vi "SubPanel_DataCollection_Rev11_v16.vi"(0 "DCPowerInformationClusterArray_Input":T8(array[cluster]), 1 "VISAPowerInfoInputArray":T5(array[cluster]), 2 "Run Data SubPanel Input":T4, 3 "RF Block Input Array":T3[](array[typedef]), 4 "Oscilloscope Info Array":T7(array[cluster]) {"vertical coupling" items=["AC", "DC", "Ground"]}, 5 "Plot Color Array":u32[](array[colorbox])=[16711686, 65351, 8978420, 14474240, 16139007, 16752640, 8958719, 16758973, 16777215, 46792, 11992992, 12961221, 16763690, 12600063, 16711835, 2953983, 40796, 13111296, 13352613, 9221011, 12964076, 12819897, 65442, 16776704, 14540253, 16740729, 10658047, 10813344, 16753521, 13413843, 8691115, 10339240, 14401205, 16746704, 7467519, 16775978, 13872558, 11387603, 13354405, 10420227, 13107364, 4060, 35208, 11817216, 7566080, 40796, 7539456, 2837073, 6372186, 7499083, 10648702, 16757152], 6 "New Run?":bool, 7 "error in":errorcluster) -> (20 "DCPowerInformationClusterArray_Output":T8(array[cluster]), 21 "VISAPowerInfoInputOutput":T5(array[cluster]), 22 "Run Data SubPanel Output":T4, 23 "RF Subpanel Output":T3[](array[typedef]), 24 "Oscilloscope Info Array":T7(array[cluster]) {"vertical coupling" items=["AC", "DC", "Ground"]}, 25 "Reinitialize?":bool, 26 "Data Was Collected?":bool, 27 "error out":errorcluster)   [LabVIEW 2019]
uses:
  Controls/DataBlockControl.ctl
  Controls/QueueDataControl_V3.ctl
  <vilib>/Utility/file.llb/Write Delimited Spreadsheet (string).vi
  <instrlib>/niScope/Acquire/Fetch/niScope Multi Fetch Binary 16.vi
  Controls/RFBlockControl.ctl
  <instrlib>/niScope/Controls/niScope vertical coupling.ctl
panel:
  out "wfm":i16[][](array[numeric])
  in  "Total Time X Min":dbl
  in  "Total Time X Max":dbl
  in  "Total Current Y Min":dbl
  in  "Total Current Y Max":dbl
  in  "Total Voltage Y Min":dbl
  in  "Total Voltage Y Max":dbl
  in  "Total Measurement Range Update":bool
  in  "Device Powered?":bool=TRUE
  out "output cluster":T2 {"vertical coupling" items=["AC", "DC", "Ground"]}
  in  "Live Measurement Range Update":bool
  in  "Live Current Y Min":dbl
  in  "Live Current Y Max":dbl
  in  "Live Voltage Y Min":dbl
  in  "Live Voltage Y Max":dbl
  out "Current Measurements Live":cluster{dbl[], dbl[]}[](graph)
  out "Voltage Measurements Live":cluster{dbl[], dbl[]}[](graph)
  out "Voltage Waveform Array":waveform(dbl)[](graph)
  out "Current Waveform Array":waveform(dbl)[](graph)
  out "Current Measurements Total":cluster{dbl[], dbl[]}[](graph)
  out "Voltage Measurements Total":cluster{dbl[], dbl[]}[](graph)
  out "Exiting":bool
  out "Full Run Information":string
  out "Ready For Next Run?":bool
  in  "Next Run":bool
  out "Recording Data":bool
  in  "Record Data Toggle":bool
  out "error of collection":errorcluster
  in  "force exit SubVI":bool
  out "RF Block Parameters Output":T3
  in  "Oscilloscope Info Array":T6(array[cluster]) {"vertical coupling" items=["AC", "DC", "Ground"]}
  out "seconds since 1Jan1904 2":timestamp
  out "seconds since 1Jan1904":timestamp
  out "Numeric 2":i32
  out "Numeric":i32
  out "RFSourceInfoArray":string[][](array[string])
  out "OscilloscopeInfoArray":string[][](array[string])
  out "DCPowerInfoArray":string[][](array[string])
  # "Background information (Important)\nThere are three sets of voltage/current graphs\n\nOne is live always and just shows what all the channels look like _______ Waveform Array\n\nOne is live when measuring and shows some duration of the recording _______ Measurements Live\n\nOne shows the entire duration of the run, but it will take a few seconds to compile, just be patient it will populate\n\n\nInstructions (More Important)"
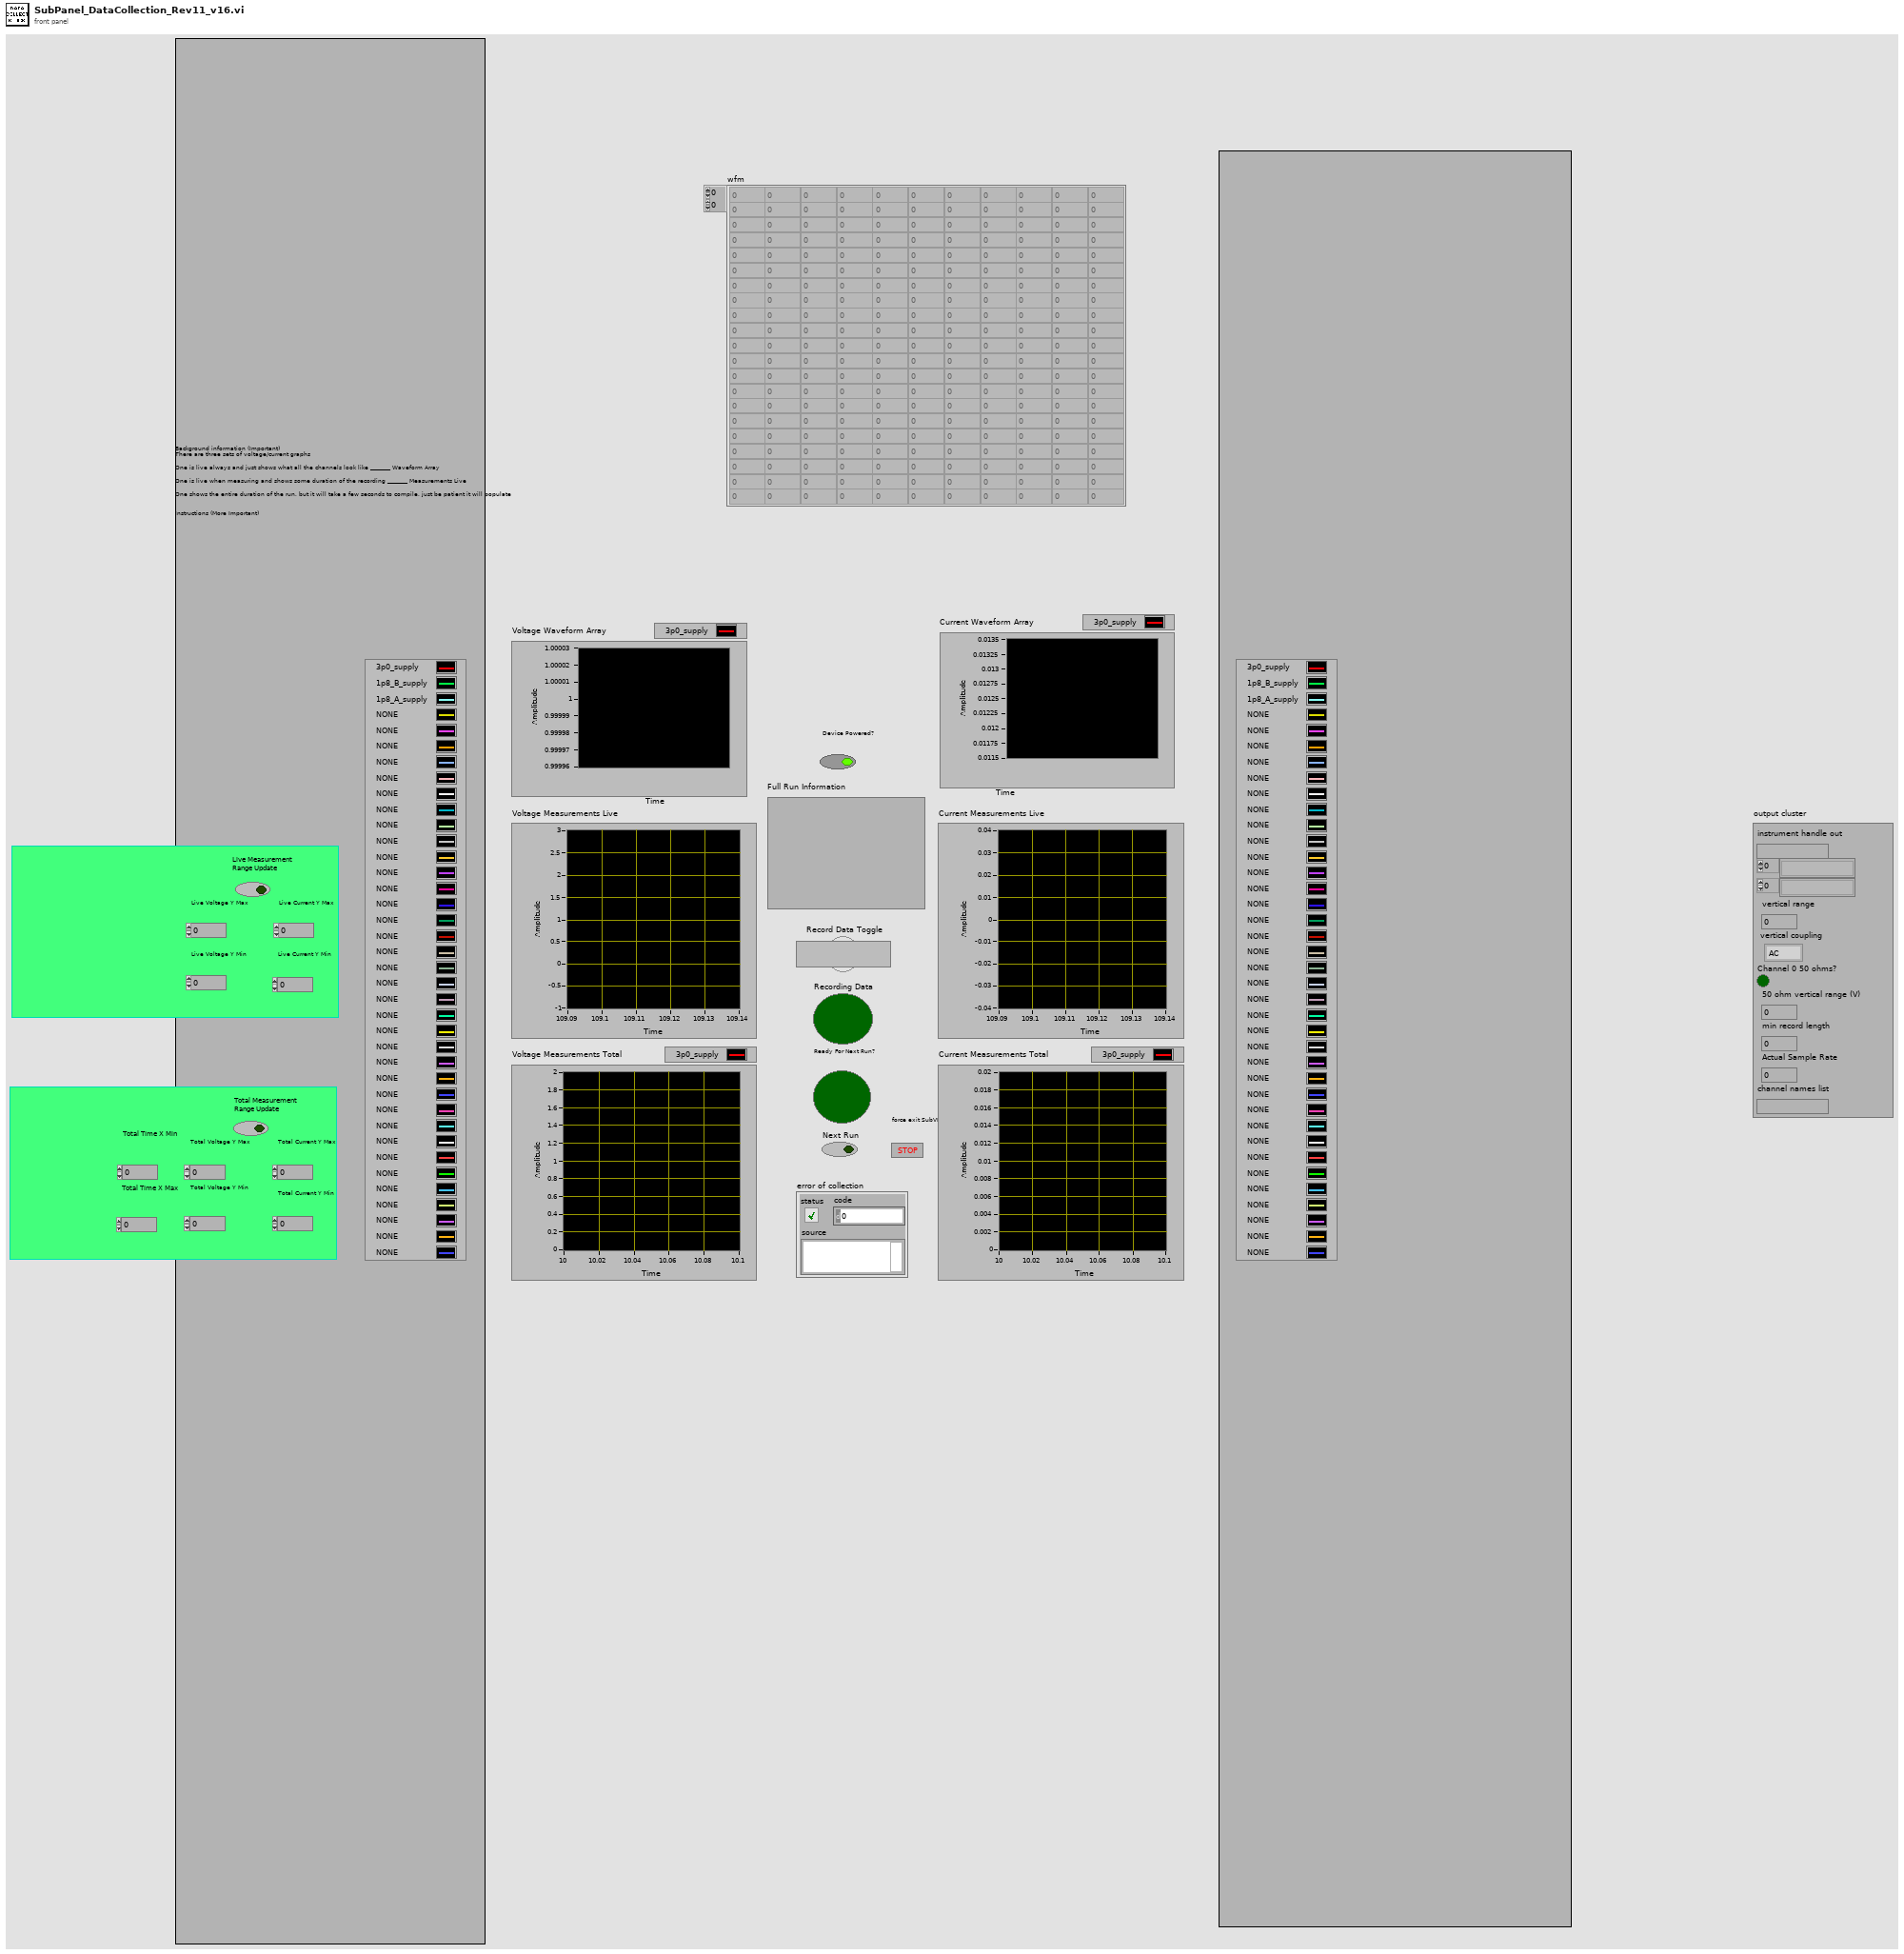
[diagram p1: front panel]
types:
  T1 = typedef "niScope vertical coupling.ctl" = i32
  T2 = cluster{"instrument handle out":refnum<k15>, string[], string[], "vertical range":dbl, "vertical coupling":T1, "Channel 0 50 ohms?":bool, "50 ohm vertical range (V)":dbl, "min record length":i32, "Actual Sample Rate":dbl, "channel names list":string}
  T3 = typedef "RFBlockControl.ctl" = cluster{"VISA resource name":refnum<visa-resource-name>, "RF Power State In":bool, "Frequency (GHz) Output":dbl, "Power (dBm) Output":dbl, "Instrument Name":string}
  T4 = typedef "DataBlockControl.ctl" = cluster{"Run Folder Parent Directory":path, "DUT":string, "Ion (ex Kr)":string, "Board Number":string, "Effective LET":string, "Test Type":enum16{"Single Event Latchup", "Single Event Transient", "Single Event Upset"}}
  T5 = cluster{"VISA resource name":refnum<visa-resource-name>, "String List":string, string[], "Input Array (Voltage,Current_Limit)":dbl[], "Input Array (Voltage,Current_Limit)":dbl[], "Channel Names":string[], "read buffer":string}[]
  T6 = cluster{"instrument handle out":refnum<k15>, "channel numbers array":string[], "channel names array":string[], "vertical range":dbl, "vertical coupling":T1, "Channel 0 50 ohms?":bool, "50 ohm vertical range (V)":dbl, "min record length":i32, "Actual Sample Rate":dbl}[]
  T7 = cluster{"instrument handle out":refnum<k15>, string[], string[], "vertical range":dbl, "vertical coupling":T1, "Channel 0 50 ohms?":bool, "50 ohm vertical range (V)":dbl, "min record length":i32, "Actual Sample Rate":dbl, "channel names list":string}[]
  T8 = cluster{"IVI Refnum out":refnum<k15>, "Active Channel Numbers String List":string, "Active Channel Numbers Array":string[], "Active Channel Voltage Array":dbl[], "Active Channel Names Array":string[], "Active Channel Current Limit Array":dbl[], "Active Channel Measure Record Delta Time Array":dbl[], "All Channel Numbers Array":string[]}[]
  T9 = typedef "QueueDataControl_V3.ctl" = cluster{"Array of fetched data":dbl[][][], "Channel Names Array":string[], "Voltage Waveform Array":waveform(dbl)[], "Current Waveform Array":waveform(dbl)[], "Resetting Time":timestamp, "Beam Logic":dbl}
  T10 = cluster{"IVI Refnum out":refnum<k15>, string, "voltage level channel 23":dbl, "Channel Name 23":string, "Current Limit":dbl, "Measure Record dt":dbl, string, "Current Threshold Reset Value Array":dbl}[]
  T11 = cluster{timestamp[], "wfm info":cluster{"actualSamples":i32, "absoluteInitialX":dbl, "relativeInitialX":dbl, "xIncrement":dbl, "offset":dbl, "gain":dbl, "reserved1":dbl, "reserved2":dbl}[][], "wfm":i16[][][]}
  T12 = cluster{"actualSamples":i32, "absoluteInitialX":dbl, "relativeInitialX":dbl, "xIncrement":dbl, "offset":dbl, "gain":dbl, "reserved1":dbl, "reserved2":dbl}[]
  T13 = cluster{"created path array":path[], "DCPowerInformationArrayOutput":cluster{"IVI Refnum out":refnum<k15>, string, "voltage level channel 23":dbl, "Channel Name 23":string, "Current Limit":dbl, "Measure Record dt":dbl, string, "Current Threshold Reset Value Array":dbl}[], string[]}
  T14 = cluster{"Array of fetched data":dbl[][], string, i32[]}
  T15 = enum16{"open", "replace", "create", "open or create", "replace or create", "replace or create with confirmation"}
  T16 = enum16{"Single Event Latchup", "Single Event Transient", "Single Event Upset"}
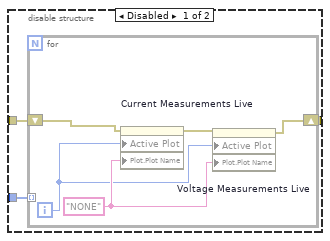
[diagram p2: hidden frame]
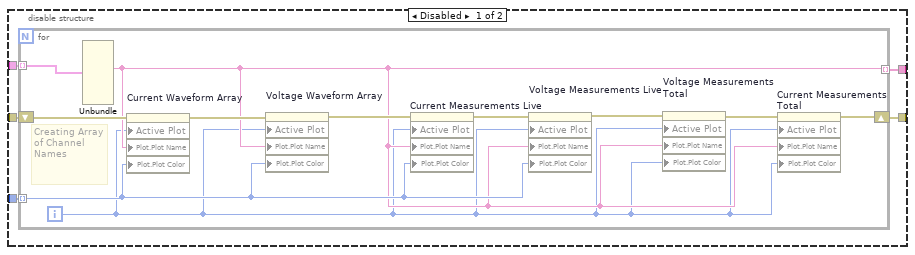
[diagram p3: hidden frame]
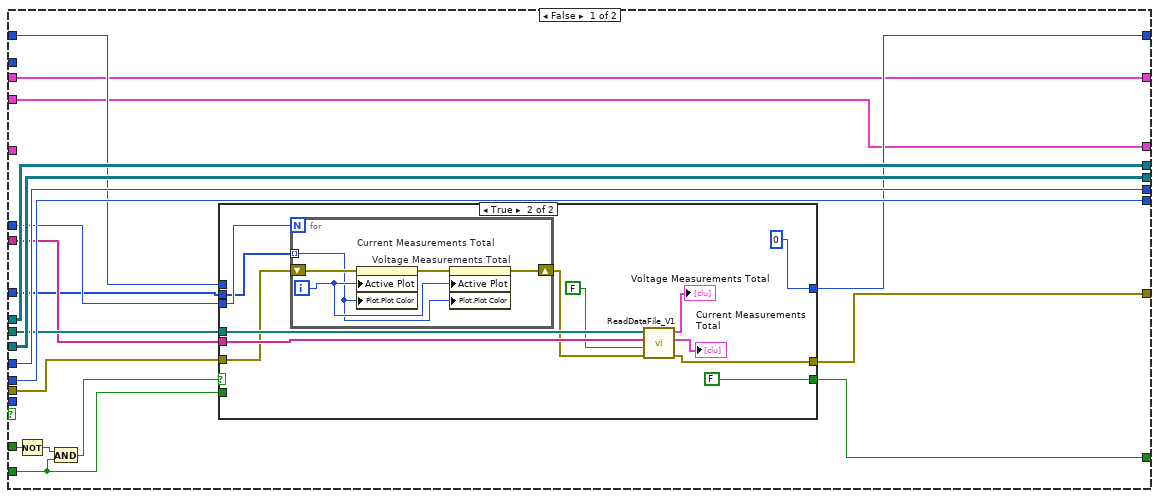
[diagram p11: hidden frame]
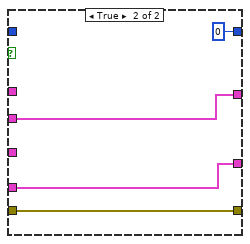
[diagram p13: hidden frame]
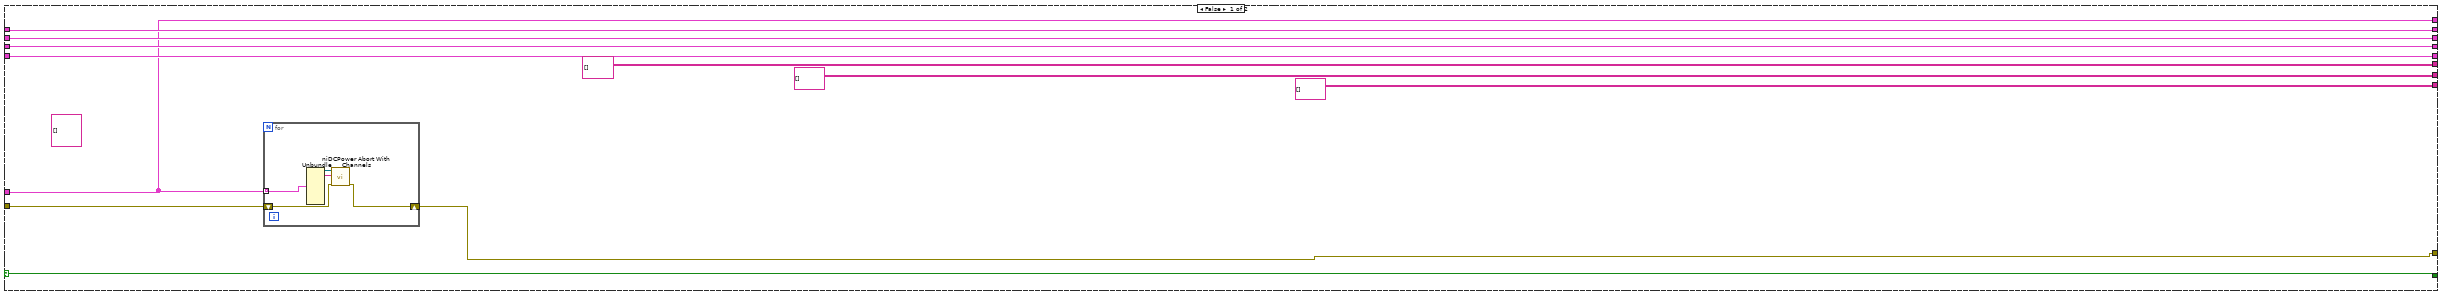
[diagram p14: hidden frame]
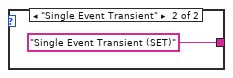
[diagram p15: hidden frame]
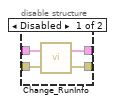
[diagram p19: hidden frame]
diagram:
  w25 = cluster{dbl[], dbl[]}[] [] ("array")
  (unwired) string[] ["Instrument Name", "Channel Name", "Instrument Channel Number", "Voltage (V)", "Current Limit (A)", "Measure Record delta Time (s)"] ("new element/subarray")
  w55 = T9 {"Array of fetched data"=[], "Channel Names Array"=[], "Voltage Waveform Array"=[], "Current Waveform Array"=[], "Resetting Time"=timestamp(0 s since 1904-01-01), "Beam Logic"=0.0} ("DCPower Queue Data Double Array Format")
  (unwired) T9 {"Array of fetched data"=[], "Channel Names Array"=[], "Voltage Waveform Array"=[], "Current Waveform Array"=[], "Resetting Time"=timestamp(0 s since 1904-01-01), "Beam Logic"=0.0} ("DCPower Double Array Queue")
  (unwired) 10000 ("binary file indexor in")
  (unwired) T4 {"Run Folder Parent Directory"=path "", "DUT"="", "Ion (ex Kr)"="", "Board Number"="", "Effective LET"="", "Test Type"=enum."Single Event Latchup"} ("Run Data Configuration")
  # "A flag to state if the devices are powered on or off"
  # "Need to make a function that will decrease the amount of loops if there are more channels active. Just exponential decay or a X/Y function but need some kind of offset which will probably be experimentally determined"
  # "Initiating the queue"
  # "echoing run information"
  # "Checking if this is a new run. If it is, a new folder is created along with references to a datafile node. If it is not new (i.e. you didn't start recording data because you needed to make a last minute change and pressed forced exit subvi), the previous folder that is theoretically empty (or just has the .txt files is used"
  # "If yes, you go into this subVI"
  # "This is the message at the beginning confirming if you want to make small changes to the program (i.e. LET)"
  # "Parameters from the configuration stage of this program"
  # "Reset the graph that is saving every 10 seconds of data. Every reset the low bound of the ten seconds is"
  # "Need to change to reflect number of channels that are being recorded. Collect this from a parameters file eventually that will be created"
  # "Indicator if the system is ready for another run. Also indicates if data was actually collected"
  # "Resets the system to start recording"
  # "A flag to ensure the warning message shows only once and doesn't lock the system"
  # "Initiating all of the DC Power instruments (doing this here so because we force abort channels in the DCPower setup because buffer overflow issues. Iterating over the instrument array and the active channel list"
  n1 = flat-sequence {
    tunnel: [w94] -> w71
    tunnel: "error in" -> [w84]
    tunnel: [w98] -> w76
    tunnel: "Run Data SubPanel Input" -> [w86]
    frame #0 {
      n2 = disable-structure shown="Enabled" {
        disable-tunnel: w84 -> [w101 w112]
        disable-tunnel: [w110 w112] -> w83
        frame Enabled {
          n3 = property on="Voltage Measurements Live" class="XYGraph (strict)"(error in=w101, "BG Color"=u32 0 ("Plot.Plot Color"), "Plot.Plot Interpolation"=u8 2) -> (error out=w100:errorcluster)  [unwired: 1 in, 1 out]
          n4 = property on="Current Measurements Live" class="XYGraph (strict)"(error in=w100, "BG Color"=u32 0 ("Plot.Plot Color"), "Plot.Plot Interpolation"=u8 2) -> (error out=w99:errorcluster)  [unwired: 1 in, 1 out]
          n5 = property on="Voltage Measurements Total" class="XYGraph (strict)"(error in=w99, "BG Color"=u32 0 ("Plot.Plot Color"), "Plot.Plot Interpolation"=u8 2) -> (error out=w111:errorcluster)  [unwired: 1 in, 1 out]
          n6 = property on="Current Measurements Total" class="XYGraph (strict)"(error in=w111, "BG Color"=u32 0 ("Plot.Plot Color"), "Plot.Plot Interpolation"=u8 2) -> (error out=w110:errorcluster)  [unwired: 1 in, 1 out]
        }
        frame Disabled {
        }
      }
      n7 = local write "Voltage Measurements Total"(cluster{dbl[], dbl[]}[] [] ("Voltage Measurements")) -> ()
      n8 = local write "Current Measurements Total"(cluster{dbl[], dbl[]}[] [] ("Current Measurements")) -> ()
      n9 = local write "Recording Data"(FALSE ("Recording Data")) -> ()
      n10 = local write "Exiting"(FALSE ("Forced Exit")) -> ()
      n11 = call "Convert_RunInfoCluster_2_RunInfoStringList.vi"("error in"=w83, "Run Number"="", "Run Data SubPanel Input"=w86) -> ("error output"=w87:errorcluster, "Run Data Output"=w88:string)
      n12 = call "Display Message to User"("error in (no error)"=w87, "Enable"=TRUE, "Message"=w88) -> ("error out"=w94:errorcluster)  [unwired: 7 in, 1 out]
      n13 = Two Button Dialog(message="Changing the LET?", 1:"No" ("F button name (\"Cancel\")"), 2:"Yes" ("T button name (\"OK\")")) -> (T button?=w98:bool)
    }
  }
  n14 = call "Convert_InstrumentReferenceArray_2_ChannelReferenceArray.vi"("error in (no error)"=w71, "DCPowerInformationClusterArray_Input"="DCPowerInformationClusterArray_Input") -> ("error out"=w70:errorcluster, "DCPowerInformationArrayOutput"=w20:T10)
  n15 = case shown="True" w76 {
    tunnel: "Run Data SubPanel Input" -> [w114 w118]
    tunnel: [w114 w117] -> w33
    tunnel: [w113 w116] -> w72
    tunnel: w70 -> [w113 w115]
    frame False {
    }
    frame True {
      n16 = disable-structure shown="Enabled" {
        disable-tunnel: w118 -> [w122 w124]
        disable-tunnel: [w121 w123] -> w117
        disable-tunnel: [w120 w126] -> w116
        disable-tunnel: w115 -> [w119 w125]
        frame Disabled {
          n17 = call "Change_RunInfo.vi"("error in (no error)"=w119, "Run Data SubPanel in"=w122) -> ("error out"=w120:errorcluster, "Run Data SubPanel out"=w121:T4)
        }
        frame Enabled {
          n18 = call "Change_RunInfo_V2.vi"("error in (no error)"=w125, "Run Data SubPanel in"=w124) -> ("error out"=w126:errorcluster, "Run Data SubPanel out"=w123:T4)
        }
      }
    }
  }
  n19 = Unbundle(w33) -> ("Run Folder Parent Directory"=w73:path)  [unwired: 5 out]
  n20 = List Folder(path=w73, error in=w72) -> (folder names=w74:string[], error out=w58:errorcluster)  [unwired: 2 in, 2 out]
  n21 = Array Size(array=w74) -> (size(s)=w61:i32)
  n22 = case shown="True" "New Run?" {
    selector: "New Run?" -> [w128 w131]
    tunnel: [w129 w133] -> w62
    tunnel: w61 -> [w129 w132]
    tunnel: [w128 w131] -> w60
    tunnel: [w127 w130] -> w59
    tunnel: w58 -> [w127 w130]
    frame False {
    }
    frame True {
      n23 = Increment(x=w132) -> (x+1=w133:i32)
    }
  }
  n24 = Number To Decimal String(number=w62) -> (decimal integer string=w65:string)  [unwired: 1 in]
  n25 = Concatenate Strings("Run_", w65) -> (w32:string)
  n26 = Array Size(array=w20) -> (size(s)=w57:i32)
  n27 = call "InitialFileFolderCreation_V2.vi"("New Run?"=w60, "error in (no error)"=w59, "Run Number"=w32, "Subfolders&NumChannelsRecorded"=w57, "base path"=w73) -> ("error out"=w31:errorcluster, "SupplementalDataFileReferenceObjectArrayWsubfolders"=w68:refnum<file>[][], "DataFileReferenceObjectArrayWsubfolders"=w69:refnum<file>[][], "created path array"=w36:path[])  [unwired: 3 in]
  n28 = call "Convert_RunInfoCluster_2_RunInfoStringList.vi"("error in"=w31, "Run Number"=w32, "Run Data SubPanel Input"=w33) -> ("error output"=w30:errorcluster, "Run Data Output"=→"Full Run Information":string)
  n29 = for {
    shift-right: [w134] -> w17
    shift-left: w30 -> [w136]
    tunnel: "DCPowerInformationClusterArray_Input" -> [w138] mode=indexing
    n30 = Unbundle(w138) -> ("IVI Refnum out"=w135:refnum<k15>, "Active Channel Numbers String List"=w137:string)  [unwired: 6 out]
    n31 = call <instrlib>:"niDCPower Initiate With Channels.vi"("error in (no error)"=w136, "channel name"=w137, "instrument handle"=w135) -> ("error out"=w134:errorcluster)  [unwired: 7 in, 1 out]
  }
  n32 = disable-structure shown="Enabled" {
    disable-tunnel: "Plot Color Array" -> [w141 _]
    disable-tunnel: [w140 w147] -> w18
    disable-tunnel: w17 -> [w139 w147]
    frame Disabled {
      n33 = for {
        shift-right: [w144] -> w140
        shift-left: w139 -> [w146]
        tunnel: w141 -> [_] mode=indexing
        i -> [w142]
        w143 = "NONE" ("Plot.Plot Name")
        n34 = property on="Current Measurements Live" class="XYGraph (strict)"(error in=w146, "Active Plot"=w142, "Plot.Plot Name"=w143) -> (error out=w145:errorcluster)  [unwired: 1 in, 1 out]
        n35 = property on="Voltage Measurements Live" class="XYGraph (strict)"(error in=w145, "Active Plot"=w142, "Plot.Plot Name"=w143) -> (error out=w144:errorcluster)  [unwired: 1 in, 1 out]
      }
    }
    frame Enabled {
    }
  }
  n36 = case shown="Error .." w18 {
    selector: w18 -> [w148 _]
    tunnel: [w148 w149] -> w3
    tunnel: w17 -> [_ w149]
    frame No Error {
    }
    frame Error {
    }
  }
  n37 = disable-structure shown="Enabled" {
    disable-tunnel: [w154 w167] -> w21
    disable-tunnel: w20 -> [w153 w168]
    disable-tunnel: "Plot Color Array" -> [w152 _]
    disable-tunnel: [w151 w166] -> w4
    disable-tunnel: w3 -> [w150 w166]
    frame Disabled {
      n38 = for {
        tunnel: w153 -> [w164] mode=indexing
        tunnel: [w156] -> w154 mode=indexing
        shift-right: [w157] -> w151
        shift-left: w150 -> [w161]
        tunnel: w152 -> [w160] mode=indexing
        i -> [w155]
        # "Creating Array of Channel Names"
        n39 = Unbundle(w164) -> ("Channel Name 23"=w156:string)  [unwired: 7 out]
        n40 = property on="Current Waveform Array" class="WFChart (strict)"(error in=w161, "Active Plot"=w155, "Plot.Plot Name"=w156, "Plot.Plot Color"=w160) -> (error out=w163:errorcluster)  [unwired: 1 in, 1 out]
        n41 = property on="Voltage Waveform Array" class="WFChart (strict)"(error in=w163, "Active Plot"=w155, "Plot.Plot Name"=w156, "Plot.Plot Color"=w160) -> (error out=w162:errorcluster)  [unwired: 1 in, 1 out]
        n42 = property on="Current Measurements Live" class="XYGraph (strict)"(error in=w162, "Active Plot"=w155, "Plot.Plot Name"=w156, "Plot.Plot Color"=w160) -> (error out=w165:errorcluster)  [unwired: 1 in, 1 out]
        n43 = property on="Voltage Measurements Live" class="XYGraph (strict)"(error in=w165, "Active Plot"=w155, "Plot.Plot Name"=w156, "Plot.Plot Color"=w160) -> (error out=w159:errorcluster)  [unwired: 1 in, 1 out]
        n44 = property on="Voltage Measurements Total" class="XYGraph (strict)"(error in=w159, "Active Plot"=w155, "Plot.Plot Name"=w156, "Plot.Plot Color"=w155) -> (error out=w158:errorcluster)  [unwired: 1 in, 1 out]
        n45 = property on="Current Measurements Total" class="XYGraph (strict)"(error in=w158, "Active Plot"=w155, "Plot.Plot Name"=w156, "Plot.Plot Color"=w155) -> (error out=w157:errorcluster)  [unwired: 1 in, 1 out]
      }
    }
    frame Enabled {
      n46 = for {
        tunnel: w168 -> [w170] mode=indexing
        tunnel: [w169] -> w167 mode=indexing
        n47 = Unbundle(w170) -> ("Channel Name 23"=w169:string)  [unwired: 7 out]
      }
    }
  }
  n48 = case shown="Error .." w4 {
    selector: w4 -> [w171 _]
    tunnel: [w171 w172] -> w2
    tunnel: w3 -> [_ w172]
    frame No Error {
    }
    frame Error {
    }
  }
  n49 = disable-structure shown="Enabled" {
    disable-tunnel: w2 -> [w176 w178]
    disable-tunnel: [w175 w178] -> w7
    disable-tunnel: [w174 _] -> w22
    disable-tunnel: w55 -> [w173 _]
    frame Enabled {
      n50 = Obtain Queue(name (unnamed)="DCPowerQueue", element data type=w173, error in (no error)=w176) -> (queue out=w174:refnum<queue>, error out=w175:errorcluster)  [unwired: 2 in, 1 out]
    }
    frame Disabled {
    }
  }
  n51 = disable-structure shown="Enabled" {
    disable-tunnel: "Oscilloscope Info Array" -> [w183 _]
    disable-tunnel: [w180 w235] -> w10
    disable-tunnel: w7 -> [w184 w235]
    frame Enabled {
      w186 = T11 {[], "wfm info"=[], "wfm"=[]} ("output cluster")
      n52 = for {
        tunnel: w183 -> [w195] mode=indexing
        shift-right: [w197] -> w185
        shift-left: w184 -> [w196]
        n53 = Unbundle By Name(w195) -> ("instrument handle out"=w194:refnum<k15>)
        n54 = call <instrlib>:"niScope Initiate Acquisition.vi"("instrument handle"=w194, "error in"=w196) -> ("error out"=w197:errorcluster)  [unwired: 12 in, 1 out]
      }
      n55 = Obtain Queue(name (unnamed)="OscilloscopeDataQueue", element data type=w186, error in (no error)=w185) -> (queue out=w187:refnum<queue>, error out=w189:errorcluster)  [unwired: 2 in, 1 out]
      n56 = while {
        shift-right: [w206] -> w181
        shift-left: w189 -> [w209]
        shift-right: [w207] -> w179
        shift-left: w183 -> [w207]
        tunnel: w187 -> [_]
        tunnel: w186 -> [w208]
        tunnel: [w205] -> _
        shift-right: [w199] -> _
        shift-left: FALSE ("x") -> [w200]
        i -> [w198]
        stop <- w204 stop-if-true
        # "BASE OFF OF TAMU POWER SCRIPTS"
        n57 = for {
          tunnel: w207 -> [w215] mode=indexing
          shift-right: [w223] -> w206
          shift-left: w209 -> [w219]
          tunnel: [w222] -> w202 mode=indexing
          tunnel: [w221] -> w201 mode=indexing
          tunnel: [w210] -> w203 mode=indexing
          shift-right: [w216] -> w199
          shift-left: w200 -> [w213]
          tunnel: w198 -> [w214]
          tunnel: w198 -> [w211]
          i -> [w220]
          n58 = Get Date/Time In Seconds() -> (seconds since 1Jan1904=w210:timestamp)
          n59 = Not(x=w213) -> (.not. x?=w218:bool)
          n60 = Unbundle By Name(w215) -> ("instrument handle out"=w227:refnum<k15>, "channel names list"=w225:string)
          n61 = And(x=w219, y=w218) -> (x .and. y?=w217:bool)
          n62 = Equal To 0?(x=w211) -> (x = 0?=w212:bool)
          n63 = case shown="True" w217 {
            tunnel: w220 -> [_ w234]
            tunnel: [w229 TRUE] -> w216
            tunnel: w215 -> [_ w233]
            tunnel: w214 -> [_ w232]
            tunnel: w213 -> [w229 _]
            tunnel: w210 -> [_ w230]
            frame False {
            }
            frame True {
              "Numeric" <- w234
              "output cluster" <- w233
              "Numeric 2" <- w232
              "seconds since 1Jan1904" <- w230
            }
          }
          n64 = case shown="True" w212 {
            tunnel: w210 -> [_ w228]
            frame False {
            }
            frame True {
              "seconds since 1Jan1904 2" <- w228
            }
          }
          n65 = call-poly <instrlib>:"niScope Fetch (poly).vi"("timeout"=0.0, "error in"=w219, "numSamples"=-1, "channels"=w225, "instrument handle"=w227) -> ("error out"=w223:errorcluster, "wfm"=w221:i16[][], "wfm info"=w222:T12)  [unwired: 3 in, 1 out]
          "wfm" <- w221
        }
        n66 = Bundle(cluster=w208, w203, "wfm info"=w202, "wfm"=w201) -> (w205:T11)
        n67 = local read "Exiting"() -> (w204:bool)
      }
      n68 = for {
        shift-right: [w192] -> w180
        shift-left: w181 -> [w193]
        tunnel: w179 -> [w191] mode=indexing
        n69 = Unbundle By Name(w191) -> ("instrument handle out"=w190:refnum<k15>)
        n70 = call <instrlib>:"niScope Abort.vi"("instrument handle"=w190, "error in"=w193) -> ("error out"=w192:errorcluster)  [unwired: 12 in, 1 out]
      }
    }
    frame Disabled {
      # "get the 1355 board"
    }
  }
  n71 = Bundle("created path array"=w36, "DCPowerInformationArrayOutput"=w20, w21) -> (w48:T13)  [unwired: 1 in]
  n72 = Array Size(array=w21) -> (size(s)=w24:i32)
  n73 = Get Date/Time In Seconds() -> (seconds since 1Jan1904=w35:timestamp)
  n74 = while {
    shift-right: [w271] -> w40
    shift-left: "DCPowerInformationClusterArray_Input" -> [w271]
    shift-right: [w275] -> w41
    shift-left: "VISAPowerInfoInputArray" -> [w275]
    shift-right: [w274] -> w43
    shift-left: w33 -> [w274]
    shift-right: [w273] -> w45
    shift-left: "RF Block Input Array" -> [w273]
    shift-right: [w272] -> w47
    shift-left: "Oscilloscope Info Array" -> [w272]
    shift-right: [w243] -> w56
    shift-left: w7 -> [w270]
    tunnel: w20 -> [w240]
    shift-right: [w269] -> _
    shift-left: FALSE -> [w266]
    tunnel: w22 -> [w268]
    shift-right: [w253] -> _
    shift-left: FALSE -> [w258]
    tunnel: [w262] -> w80
    shift-right: [w256] -> _
    shift-left: TRUE ("x .and. y?") -> [w257]
    shift-right: [w254] -> _
    shift-left: w35 -> [w255]
    tunnel: [w253] -> w39
    tunnel: w55 -> [w251]
    shift-right: [w248] -> w14
    shift-left: timestamp(0 s since 1904-01-01) ("seconds since 1Jan1904") -> [w247]
    shift-right: [w237] -> _
    shift-left: TRUE -> [w236]
    stop <- w252 stop-if-true
    # "If I am going to reset the entire configuration or if we are going up in LET only. True, reset the system. False, don't reset the system"
    n75 = Not(x=w258) -> (.not. x?=w260:bool)
    n76 = And(x="Record Data Toggle", y=w260) -> (x .and. y?=w261:bool)
    "Recording Data" <- w261
    n77 = case shown="False" w261 {
      tunnel: w240 -> [w343 w358]
      tunnel: w270 -> [w341 w365]
      tunnel: [w331 w353] -> w250
      tunnel: [w332 w352] -> w249
      tunnel: w266 -> [_ w363]
      tunnel: [FALSE w364] -> w269
      tunnel: w268 -> [_ w362]
      tunnel: [w330 w361] -> w242
      tunnel: "Record Data Toggle" -> [w338 _]
      tunnel: w258 -> [w339 _]
      tunnel: w257 -> [w334 _]
      tunnel: [w335 TRUE] -> w256
      tunnel: w255 -> [w333 w366]
      tunnel: [w333 w356] -> w254
      tunnel: w251 -> [_ w360]
      tunnel: [w329 w350] -> w248
      tunnel: w247 -> [w329 w349]
      frame False {
        n78 = And(x=w338, y=w339) -> (x .and. y?=w337:bool)
        n79 = And(x=w334, y=w337) -> (x .and. y?=w336:bool)
        n80 = case shown="True" w336 {
          tunnel: [w345 w347] -> w340
          tunnel: w341 -> [w345 w348]
          tunnel: [w344 FALSE] -> w335
          tunnel: w334 -> [w344 _]
          frame False {
          }
          frame True {
            n81 = call "Display Message to User2"("error in (no error)"=w348) -> ("error out"=w347:errorcluster)  [unwired: 9 in, 1 out]
          }
        }
        n82 = call "Fetch&Process_Measurements_V4.vi"("DCPowerInformation_byChannel"=w343, "Initial Time"=w333, "error in (no error)"=w340) -> ("Current Waveform Array"=w331:waveform(dbl)[], "Voltage Waveform Array"=w332:waveform(dbl)[], "error out"=w330:errorcluster)  [unwired: 6 in, 4 out]
      }
      frame True {
        n83 = case shown="False" w363 {
          tunnel: [w368 w374] -> w356
          tunnel: w366 -> [_ w374]
          tunnel: w365 -> [w369 w373]
          tunnel: [w369 w373] -> w357
          tunnel: [TRUE w372] -> w364
          tunnel: w363 -> [_ w372]
          tunnel: [w368 w371] -> w350
          tunnel: w349 -> [_ w371]
          frame False {
            n84 = Get Date/Time In Seconds() -> (seconds since 1Jan1904=w368:timestamp)
          }
          frame True {
          }
        }
        n85 = call "Fetch&Process_Measurements_V4.vi"("DCPowerInformation_byChannel"=w358, "Initial Time"=w356, "error in (no error)"=w357) -> ("Data As dbl Array"=w355:dbl[][][], "Channel Number Array"=w354:string[], "Current Waveform Array"=w353:waveform(dbl)[], "Voltage Waveform Array"=w352:waveform(dbl)[], "error out"=w351:errorcluster)  [unwired: 6 in, 2 out]
        n86 = Bundle(cluster=w360, "Array of fetched data"=w355, "Channel Names Array"=w354) -> (w359:T9)  [unwired: 4 in]
        n87 = Enqueue Element(queue=w362, element=w359, error in (no error)=w351) -> (error out=w361:errorcluster)  [unwired: 1 in, 2 out]
      }
    }
    "Current Waveform Array" <- w250
    "Voltage Waveform Array" <- w249
    n88 = Not(x=w261) -> (.not. x?=w267:bool)
    n89 = And(x=w267, y=w266) -> (x .and. y?=w265:bool)
    n90 = Exclusive Or(1:"Device Powered?", 2:w236) -> (0:w239:bool)
    n91 = case shown="False" w239 {
      tunnel: [w277 w281] -> w241
      tunnel: w242 -> [w277 w280]
      tunnel: w240 -> [_ w282]
      tunnel: "Device Powered?" -> [w276 w279]
      tunnel: [w276 w278] -> w237
      frame False {
      }
      frame True {
        n92 = case shown="True" w279 {
          selector: w279 -> [w283 w299]
          tunnel: w282 -> [w286 w302]
          tunnel: [w284 w301] -> w281
          tunnel: w280 -> [w285 w300]
          tunnel: [w283 w299] -> w278
          frame False {
            n93 = for {
              tunnel: w286 -> [w298] mode=indexing
              shift-right: [w288] -> w284
              shift-left: w285 -> [w289]
              n94 = Unbundle(w298) -> ("IVI Refnum out"=w297:refnum<k15>, w290:string)  [unwired: 6 out]
              n95 = call <instrlib>:"niDCPower Abort With Channels.vi"("error in (no error)"=w289, "channel name"=w290, "instrument handle"=w297) -> ("error out"=w296:errorcluster, "instrument handle out"=w295:refnum<k15>)  [unwired: 7 in]
              n96 = call <instrlib>:"niDCPower Configure Voltage Level.vi"("error in (no error)"=w296, "voltage level"=0.0, "channel name"=w290, "instrument handle"=w295) -> ("error out"=w294:errorcluster, "instrument handle out"=w293:refnum<k15>)  [unwired: 6 in]
              n97 = call <instrlib>:"niDCPower Commit With Channels.vi"("error in (no error)"=w294, "channel name"=w290, "instrument handle"=w293) -> ("error out"=w292:errorcluster, "instrument handle out"=w291:refnum<k15>)  [unwired: 7 in]
              n98 = call <instrlib>:"niDCPower Initiate With Channels.vi"("error in (no error)"=w292, "channel name"=w290, "instrument handle"=w291) -> ("error out"=w288:errorcluster)  [unwired: 7 in, 1 out]
            }
          }
          frame True {
            n99 = for {
              tunnel: w302 -> [w314] mode=indexing
              shift-right: [w304] -> w301
              shift-left: w300 -> [w305]
              n100 = Unbundle(w314) -> ("IVI Refnum out"=w313:refnum<k15>, w306:string, "voltage level channel 23"=w303:dbl)  [unwired: 5 out]
              n101 = call <instrlib>:"niDCPower Abort With Channels.vi"("error in (no error)"=w305, "channel name"=w306, "instrument handle"=w313) -> ("error out"=w312:errorcluster, "instrument handle out"=w311:refnum<k15>)  [unwired: 7 in]
              n102 = call <instrlib>:"niDCPower Configure Voltage Level.vi"("error in (no error)"=w312, "voltage level"=w303, "channel name"=w306, "instrument handle"=w311) -> ("error out"=w310:errorcluster, "instrument handle out"=w309:refnum<k15>)  [unwired: 6 in]
              n103 = call <instrlib>:"niDCPower Commit With Channels.vi"("error in (no error)"=w310, "channel name"=w306, "instrument handle"=w309) -> ("error out"=w308:errorcluster, "instrument handle out"=w307:refnum<k15>)  [unwired: 7 in]
              n104 = call <instrlib>:"niDCPower Initiate With Channels.vi"("error in (no error)"=w308, "channel name"=w306, "instrument handle"=w307) -> ("error out"=w304:errorcluster)  [unwired: 7 in, 1 out]
            }
          }
        }
      }
    }
    n105 = case shown="True" w265 {
      tunnel: w241 -> [w325 w327]
      tunnel: [w326 TRUE] -> w253
      tunnel: w258 -> [w326 _]
      tunnel: [w325 w327] -> w243
      frame False {
      }
      frame True {
      }
    }
    "error of collection" <- w243
    "Ready For Next Run?" <- w253
    n106 = And(x="Next Run", y=w253) -> (x .and. y?=w264:bool)
    n107 = Or(x="force exit SubVI", y=w264) -> (x .or. y?=w245:bool)
    n108 = Or(x=w243, y=w245) -> (x .or. y?=w244:bool)
    n109 = case shown="True" w244 {
      selector: w244 -> [w316 _]
      tunnel: w243 -> [_ w319]
      tunnel: [w316 TRUE] -> w252
      tunnel: [TRUE ("T button?") w317] -> w262
      frame False {
        # "Don't end the run"
      }
      frame True {
        n110 = case shown="Error .." w319 {
          tunnel: [w320 TRUE] -> w317
          frame No Error {
            # "Option to continue the run as is or reset for a new configuration"
            n111 = Two Button Dialog(message="Would you like to change parameters before the next run? ( you will have an option to change LET and board number regardless) ", 1:"No, I may only want to change LET or board number" ("F button name (\"Cancel\")"), 2:"Yes, I want to make changes " ("T button name (\"OK\")")) -> (T button?=w320:bool)
          }
          frame Error {
            # "End the run immediately. There is an error or an immediate issue with the VI"
          }
        }
      }
    }
    "Exiting" <- w252
  }
  "Reinitialize?" <- w80
  n112 = while {
    tunnel: w22 -> [w414]
    shift-right: [w375] -> w8
    shift-left: w7 -> [w413]
    tunnel: w36 -> [w410]
    shift-right: [w403] -> w54
    shift-left: w69 -> [w411]
    shift-right: [w402] -> w53
    shift-left: w68 -> [w409]
    shift-right: [w405] -> _
    shift-left: 0 ("binary file indexor in") -> [w408]
    shift-right: [w404] -> _
    shift-left: 0 ("binary file indexor in") -> [w407]
    tunnel: 1000 ("binary file indexor in") -> [w406]
    tunnel: w21 -> [w412]
    tunnel: w24 -> [w381]
    shift-right: [w391] -> _
    shift-left: FALSE -> [w390]
    shift-right: [w387] -> _
    shift-left: 0 -> [w388]
    shift-right: [w386] -> _
    shift-left: w25 -> [w383]
    shift-right: [w385] -> _
    shift-left: w25 -> [w384]
    tunnel: 251 ("y") -> [w382]
    tunnel: "Plot Color Array" -> [w380]
    stop <- w399 stop-if-true
    # "If recording data is on, there should always be elements in the queue, so I shouldn't have to worry about a state where the \"recording data\" is active but there is no data in the queue, if so, then I'll just have to find an alternative to the OR statement"
    n113 = Get Queue Status(queue=w414, error in (no error)=w413) -> (queue out=w396:refnum<queue>, error out=w397:errorcluster, # elements in queue=w392:i32)  [unwired: 1 in, 5 out]
    n114 = local read "Recording Data"() -> (w389:bool)
    n115 = Flush Queue(queue=w396, error in (no error)=w397) -> (remaining elements=w395:T9[], error out=w398:errorcluster)  [unwired: 1 out]
    n116 = Not Equal To 0?(x=w392) -> (x != 0?=w394:bool)
    n117 = And(x=w394, y=w389) -> (x .and. y?=w393:bool)
    n118 = case shown="True" w393 {
      tunnel: w395 -> [_ w506]
      tunnel: w398 -> [w444 w500]
      tunnel: w412 -> [w445 w493]
      tunnel: w411 -> [w452 w505]
      tunnel: w410 -> [w446 w504]
      tunnel: w409 -> [w453 w503]
      tunnel: w408 -> [w451 w502]
      tunnel: w407 -> [w450 w492]
      tunnel: w406 -> [_ w491]
      tunnel: [w451 w499] -> w405
      tunnel: [w450 w498] -> w404
      tunnel: [w452 w495] -> w403
      tunnel: [w453 w494] -> w402
      tunnel: [w443 w485] -> w379
      tunnel: [w442 TRUE] -> w391
      tunnel: w390 -> [w441 _]
      tunnel: w389 -> [w449 _]
      tunnel: w388 -> [w440 w483]
      tunnel: [w439 w482] -> w387
      tunnel: [w438 w489] -> w386
      tunnel: [w437 w486] -> w385
      tunnel: w384 -> [w437 w481]
      tunnel: w383 -> [w438 w480]
      tunnel: w382 -> [_ w474]
      tunnel: w381 -> [w436 _]
      tunnel: w380 -> [w435 _]
      frame False {
        n119 = Not(x=w449) -> (.not. x?=w448:bool)
        n120 = And(x=w448, y=w441) -> (x .and. y?=w447:bool)
        n121 = case shown="True" w447 {
          tunnel: w446 -> [_ w468]
          tunnel: w445 -> [_ w467]
          tunnel: w444 -> [w456 w460]
          tunnel: [w456 w465] -> w443
          tunnel: [w455 FALSE] -> w442
          tunnel: w441 -> [w455 _]
          tunnel: w440 -> [w454 _]
          tunnel: [w454 0] -> w439
          tunnel: w436 -> [_ w458]
          tunnel: w435 -> [_ w457]
          frame False {
          }
          frame True {
            n122 = for {
              N: w458 -> [_]
              shift-right: [w471] -> w459
              shift-left: w460 -> [w472]
              tunnel: w457 -> [w469] mode=indexing
              i -> [w470]
              n123 = property on="Current Measurements Total" class="XYGraph (strict)"(error in=w472, "Active Plot"=w470, "Plot.Plot Color"=w469) -> (error out=w473:errorcluster)  [unwired: 1 in, 1 out]
              n124 = property on="Voltage Measurements Total" class="XYGraph (strict)"(error in=w473, "Active Plot"=w470, "Plot.Plot Color"=w469) -> (error out=w471:errorcluster)  [unwired: 1 in, 1 out]
            }
            n125 = call "ReadDataFile_V1.vi"("error in (no error)"=w459, "Create CSV files?"=FALSE, "Channel Names Array"=w467, "DataFolder Path"=w468) -> ("error out"=w465:errorcluster, "Current Measurements"=→"Current Measurements Total":cluster{dbl[], dbl[]}[], "Voltage Measurements"=→"Voltage Measurements Total":cluster{dbl[], dbl[]}[])  [unwired: 5 in]
          }
        }
      }
      frame True {
        # "structure where each channel has its own data and supplemental file. Intent for faster data reading speeds in post processing. Probably not since would be i^3, but if we used multiple cores, maybe it would be advantageous"
        n126 = call "FilePathCreation_DCPower_V2.vi"("binary file input reference array 1"=w505, "Channel Name Input array"=w493, "data output directory folder"=w504, "binary file indexor in"=w502, "Reset counter in"=w492, "error in (no error)"=w500, "binary file input reference array 2"=w503, "reset threshold"=w491) -> ("binary file output reference array"=w497:refnum<file>[], "binary file output reference array 2"=w496:refnum<file>[], "binary file indexor out"=w499:i32, "reset counter out"=w498:i32, "error out"=w501:errorcluster)  [unwired: 3 in]
        n127 = for {
          shift-right: [w553] -> w484
          shift-left: w501 -> [w554]
          tunnel: w506 -> [w563]
          tunnel: w496 -> [w560] mode=indexing
          tunnel: w497 -> [w559] mode=indexing
          tunnel: [w558] -> w494 mode=indexing
          tunnel: [w552] -> w495 mode=indexing
          tunnel: [w541] -> w488 mode=indexing
          tunnel: [w540] -> w487 mode=indexing
          i -> [w557]
          n128 = for {
            tunnel: w563 -> [w576] mode=indexing
            tunnel: w557 -> [w573]
            tunnel: [w568] -> w548 mode=concatenating
            tunnel: [w572] -> w562
            tunnel: w560 -> [w571]
            tunnel: w559 -> [w569]
            tunnel: [w569] -> w555
            tunnel: [w571] -> w558
            tunnel: [w570] -> w561 mode=concatenating
            n129 = Unbundle(w576) -> ("Array of fetched data"=w575:dbl[][][], "Channel Names Array"=w574:string[])  [unwired: 4 out]
            n130 = Index Array(array=w574, index=w573) -> (element=w572:string)
            n131 = Index Array(array=w575, index (dim 0)=w573) -> (element=w568:dbl[][])  [unwired: 2 in]
            n132 = Array Size(array=w568) -> (size(s)=w570:i32[])
          }
          n133 = Bundle("Array of fetched data"=w548, w562, w561) -> (w556:T14)  [unwired: 1 in]
          n134 = Index Array(array=w548, index (row)=2) -> (element=w545:dbl[])  [unwired: 1 in]
          n135 = Index Array(array=w548, index (row)=1) -> (element=w546:dbl[])  [unwired: 1 in]
          n136 = Index Array(array=w548, index (row)=0) -> (element=w547:dbl[])  [unwired: 1 in]
          n137 = call "DataFileNode_Entry_V4.vi"("error in (no error)"=w554, "Queued Elements"=w556, "Byte Stream File in"=w555) -> ("error out"=w553:errorcluster, "Byte Stream File out"=w552:refnum<file>)  [unwired: 7 in]
          n138 = for {
            tunnel: [w565] -> w544 mode=indexing if=w564
            tunnel: w547 -> [w565] mode=indexing
            tunnel: [w567] -> w542 mode=indexing if=w564
            tunnel: w546 -> [w567] mode=indexing
            tunnel: [w566] -> w543 mode=indexing if=w564
            tunnel: w545 -> [w566] mode=indexing
            n139 = Not Equal To 0?(x=w565) -> (x != 0?=w564:bool)
          }
          n140 = Bundle(w544, w542) -> (w541:cluster{dbl[], dbl[]})  [unwired: 1 in]
          n141 = Bundle(w544, w543) -> (w540:cluster{dbl[], dbl[]})  [unwired: 1 in]
        }
        n142 = Greater?(x=w483, y=w474) -> (0:w476:bool)
        n143 = Array Size(array=w480) -> (size(s)=w479:i32)
        n144 = Equal?(x=w479, y=0) -> (x = y?=w477:bool)
        n145 = Or(x=w476, y=w477) -> (x .or. y?=w475:bool)
        n146 = case shown="False" w475 {
          tunnel: [w512 w536] -> w489
          tunnel: w480 -> [w516 _]
          tunnel: w488 -> [w515 w536]
          tunnel: w481 -> [w514 _]
          tunnel: w487 -> [w513 w537]
          tunnel: [w511 w537] -> w486
          tunnel: [w510 w539] -> w485
          tunnel: w484 -> [w509 w539]
          tunnel: w483 -> [w508 _]
          tunnel: [w507 0] -> w482
          frame False {
            n147 = for {
              tunnel: w516 -> [w535] mode=indexing
              tunnel: w515 -> [w532] mode=indexing
              tunnel: w514 -> [w529] mode=indexing
              tunnel: w513 -> [w528] mode=indexing
              tunnel: [w519] -> w512 mode=indexing
              tunnel: [w518] -> w511 mode=indexing
              shift-right: [w517] -> w510
              shift-left: w509 -> [w517]
              n148 = Unbundle(w535) -> (w534:dbl[], w533:dbl[])
              n149 = Unbundle(w532) -> (w531:dbl[], w530:dbl[])
              n150 = Unbundle(w529) -> (w527:dbl[], w526:dbl[])
              n151 = Unbundle(w528) -> (w525:dbl[], w524:dbl[])
              n152 = Insert Into Array(array=w527, new element=w525) -> (w522:dbl[])  [unwired: 1 in]
              n153 = Insert Into Array(array=w534, new element=w531) -> (w520:dbl[])  [unwired: 1 in]
              n154 = Insert Into Array(array=w526, new element=w524) -> (w523:dbl[])  [unwired: 1 in]
              n155 = Insert Into Array(array=w533, new element=w530) -> (w521:dbl[])  [unwired: 1 in]
              n156 = Bundle(w522, w523) -> (w518:cluster{dbl[], dbl[]})  [unwired: 1 in]
              n157 = Bundle(w520, w521) -> (w519:cluster{dbl[], dbl[]})  [unwired: 1 in]
            }
            n158 = Increment(x=w508) -> (x+1=w507:i32)
          }
          frame True {
          }
        }
        "Voltage Measurements Live" <- w489
        "Current Measurements Live" <- w486
      }
    }
    n159 = Equal To 0?(x=w392) -> (x = 0?=w400:bool)
    n160 = case shown="True" "Live Measurement Range Update" {
      tunnel: w379 -> [w425 w434]
      tunnel: [w425 w433] -> w376
      frame False {
      }
      frame True {
        (unwired) 0.001 ("Delay Time (s)")
        n161 = property on="Voltage Measurements Live" class="XYGraph (strict)"(error in=w434, "YScale.Maximum"="Live Voltage Y Max", "YScale.Minimum"="Live Voltage Y Min") -> (error out=w427:errorcluster)  [unwired: 1 in, 1 out]
        n162 = property on="Current Measurements Live" class="XYGraph (strict)"(error in=w427, "ActXScl"=0 ("Active X Scale")) -> (error out=w426:errorcluster)  [unwired: 1 in, 1 out]
        n163 = property on="Current Measurements Live" class="XYGraph (strict)"(error in=w426, "YScale.Maximum"="Live Current Y Max", "YScale.Minimum"="Live Current Y Min") -> (error out=w433:errorcluster)  [unwired: 1 in, 1 out]
      }
    }
    n164 = local read "Exiting"() -> (w401:bool)
    n165 = And(x=w400, y=w401) -> (x .and. y?=w399:bool)
    n166 = case shown="True" "Total Measurement Range Update" {
      tunnel: w376 -> [w415 w424]
      tunnel: [w415 w422] -> w375
      frame False {
      }
      frame True {
        n167 = property on="Voltage Measurements Total" class="XYGraph (strict)"(error in=w424, "YScale.Maximum"="Total Voltage Y Max", "YScale.Minimum"="Total Voltage Y Min", "XScale.Maximum"="Total Time X Max", "XScale.Minimum"="Total Time X Min") -> (error out=w423:errorcluster)  [unwired: 1 in, 1 out]
        n168 = property on="Current Measurements Total" class="XYGraph (strict)"(error in=w423, "YScale.Maximum"="Total Current Y Max", "YScale.Minimum"="Total Current Y Min", "XScale.Maximum"="Total Time X Max", "XScale.Minimum"="Total Time X Min") -> (error out=w422:errorcluster)  [unwired: 1 in, 1 out]
      }
    }
  }
  n169 = Merge Errors(w8, w10) -> (w9:errorcluster)
  n170 = for {
    tunnel: w54 -> [w581] mode=indexing
    tunnel: w53 -> [w579] mode=indexing
    shift-right: [w577] -> w52
    shift-left: w9 -> [w580]
    n171 = Close File(refnum=w581, error in=w580) -> (error out=w578:errorcluster)  [unwired: 1 out]
    n172 = Close File(refnum=w579, error in=w578) -> (error out=w577:errorcluster)  [unwired: 1 out]
  }
  n173 = Merge Errors(w56, w52) -> (w49:errorcluster)
  n174 = Unbundle(w48) -> ("created path array"=w16:path[])  [unwired: 2 out]
  n175 = case shown="True" w39 {
    selector: w39 -> [w588 w728]
    tunnel: w49 -> [w583 w734]
    tunnel: [w592 w666] -> w11
    tunnel: w47 -> [w592 w733]
    tunnel: [w591 w668] -> w46
    tunnel: w45 -> [w591 w732]
    tunnel: [w590 w654] -> w44
    tunnel: w43 -> [w590 w731]
    tunnel: [w589 w671] -> w42
    tunnel: w41 -> [w589 w730]
    tunnel: [w584 w673] -> w5
    tunnel: w40 -> [w584 w729]
    tunnel: [w588 w728] -> w38
    tunnel: [string[][] [] ("DCPowerInfoArray") w664] -> w37
    tunnel: w16 -> [_ w599]
    tunnel: [string[][] [] ("DCPowerInfoArray") w662] -> w12
    tunnel: [string[][] [] ("DCPowerInfoArray") w656] -> w27
    tunnel: [w582 w601] -> w15
    tunnel: w14 -> [_ w600]
    frame False {
      (unwired) string[][][] []
      n176 = for {
        tunnel: w584 -> [w595] mode=indexing
        shift-right: [w596] -> w582
        shift-left: w583 -> [w597]
        n177 = Unbundle(w595) -> ("IVI Refnum out"=w594:refnum<k15>, "Active Channel Numbers String List"=w593:string)  [unwired: 6 out]
        n178 = call <instrlib>:"niDCPower Abort With Channels.vi"("error in (no error)"=w597, "channel name"=w593, "instrument handle"=w594) -> ("error out"=w596:errorcluster)  [unwired: 7 in, 1 out]
      }
    }
    frame True {
      # "This will be indexed eventually"
      n179 = for {
        shift-right: [w828] -> w598
        shift-left: w734 -> [w839]
        tunnel: w729 -> [w826] mode=indexing
        shift-right: [w838] -> w704
        shift-left: w733 -> [w838]
        shift-right: [w837] -> w703
        shift-left: w732 -> [w837]
        shift-right: [w836] -> w702
        shift-left: w731 -> [w836]
        shift-right: [w835] -> w701
        shift-left: w730 -> [w835]
        shift-right: [w834] -> w700
        shift-left: w729 -> [w834]
        shift-right: [w832] -> w705
        shift-left: string[][] [] ("DCPowerInfoArray") -> [w833]
        # "This puts all the instruments together in one output"
        n180 = Unbundle(w826) -> ("IVI Refnum out"=w841:refnum<k15>, "Active Channel Numbers String List"=w840:string)  [unwired: 6 out]
        n181 = call <instrlib>:"niDCPower Abort With Channels.vi"("error in (no error)"=w839, "channel name"=w840, "instrument handle"=w841) -> ("error out"=w829:errorcluster)  [unwired: 7 in, 1 out]
        n182 = call "DCPower_ParameterCreation.vi"("error in"=w829, "Precision"="8", "DCPowerInformationByInstrument"=w826) -> ("error out"=w828:errorcluster, "DCPowerInfoArray"=w827:string[][])
        n183 = Insert Into Array(array=w833, index (col)=0 ("disabled index (col)"), new element=w827) -> (w832:string[][])  [unwired: 1 in]
      }
      n184 = Concatenate Strings("Channel Name " ("string")) -> (w717:string)
      n185 = Concatenate Strings("Voltage (V) " ("string")) -> (w719:string)
      n186 = Concatenate Strings("Measure Record delta Time (s) " ("string")) -> (w721:string)
      n187 = Concatenate Strings("Instrument Name " ("string")) -> (w716:string)
      n188 = Concatenate Strings("Instrument Channel Number " ("string")) -> (w718:string)
      n189 = Concatenate Strings("Current Limit (A) " ("string")) -> (w720:string)
      n190 = Build Array(w716, w717, w718, w719, w720, w721) -> (w709:string[])
      n191 = Build Path(base path=w599, name or relative path="DCPOW_Params.csv") -> (appended path=w724:path)
      n192 = Insert Into Array(array=w705, index (col)=0 ("disabled index (col)"), new element=w709) -> (w708:string[][])  [unwired: 1 in]
      n193 = call-poly <vilib>:"Write Delimited Spreadsheet.vi"("file path (dialog if empty)"=w724, "format (%s)"="%s" ("format (%.3f)"), "2D data"=w708, "error in (no error)"=w598, "transpose? (no:F)"=TRUE, "delimiter (\\t)"="," ("delimiter (\\t)")) -> ("error out"=w706:errorcluster)  [unwired: 8 in, 1 out]
      n194 = for {
        shift-right: [w820] -> w686
        shift-left: w706 -> [w820]
        shift-right: [w815] -> w674
        shift-left: w700 -> [w815]
        shift-right: [w816] -> w672
        shift-left: w701 -> [w816]
        shift-right: [w817] -> w670
        shift-left: w702 -> [w817]
        shift-right: [w818] -> w669
        shift-left: w703 -> [w818]
        shift-right: [w819] -> w665
        shift-left: w705 -> [w819]
        tunnel: w704 -> [w814] mode=indexing
        tunnel: [w814] -> w667 mode=indexing
        shift-right: [w783] -> w663
        shift-left: string[][] [] ("DCPowerInfoArray") -> [w789]
        n195 = Unbundle(w814) -> ("instrument handle out"=w813:refnum<k15>, w786:string[], w787:string[], "vertical range"=w808:dbl, "vertical coupling"=w802:T1, "Channel 0 50 ohms?"=w807:bool, "50 ohm vertical range (V)"=w806:dbl, "min record length"=w801:i32, "Actual Sample Rate"=w800:dbl)  [unwired: 1 out]
        n196 = Array Size(array=w786) -> (size(s)=w809:i32)
        n197 = Initialize Array(w808, w809) -> (w805:dbl[])
        n198 = Decimal String To Number(string="8") -> (number=w784:i32)  [unwired: 2 in, 1 out]
        n199 = case shown="True" w807 {
          tunnel: w806 -> [_ w823]
          tunnel: w805 -> [w821 w825]
          tunnel: [w821 w822] -> w804
          frame False {
          }
          frame True {
            n200 = Replace Array Subset(array=w825, new element=w823, index=0) -> (w822:dbl[])
          }
        }
        n201 = Number To Fractional String(number=w800, precision (6)=w784) -> (F-format string=w794:string)  [unwired: 2 in]
        n202 = Number To Decimal String(number=w801) -> (decimal integer string=w795:string)  [unwired: 1 in]
        n203 = Concatenate Strings(w813) -> (w811:string)
        n204 = Number To Fractional String(number=w804, precision (6)=w784) -> (F-format string=w803:string[])  [unwired: 2 in]
        n205 = Number To Decimal String(number=w802) -> (decimal integer string=w796:string)  [unwired: 1 in]
        n206 = Array Size(array=w786) -> (size(s)=w812:i32)
        n207 = Initialize Array(w811, w812) -> (w810:string[])
        n208 = Array Size(array=w786) -> (size(s)=w799:i32)
        n209 = Array Size(array=w786) -> (size(s)=w797:i32)
        n210 = Array Size(array=w786) -> (size(s)=w798:i32)
        n211 = Initialize Array(w796, w799) -> (w793:string[])
        n212 = Initialize Array(w794, w797) -> (w791:string[])
        n213 = Initialize Array(w795, w798) -> (w792:string[])
        n214 = Build Array(w810, w787, w786, w803, w793, w792, w791) -> (w788:string[][])
        n215 = Insert Into Array(array=w789, index (col)=0 ("disabled index (col)"), new element=w788) -> (w783:string[][])  [unwired: 1 in]
      }
      n216 = Build Array("Instrument Name " ("string"), "Channel Name" ("element"), "Instrument Channel Number" ("element"), "Vertical Range (V)" ("element"), "Vertical Coupling" ("element"), "Min Record Length" ("element"), "Actual Sample Rate" ("element")) -> (w690:string[])
      n217 = Insert Into Array(array=w663, index (col)=0 ("disabled index (col)"), new element=w690) -> (w683:string[][])  [unwired: 1 in]
      n218 = Build Path(base path=w599, name or relative path="Oscilloscope_Params.csv") -> (appended path=w688:path)
      n219 = call-poly <vilib>:"Write Delimited Spreadsheet.vi"("file path (dialog if empty)"=w688, "format (%s)"="%s" ("format (%.3f)"), "2D data"=w683, "error in (no error)"=w686, "transpose? (no:F)"=TRUE, "delimiter (\\t)"="," ("delimiter (\\t)")) -> ("error out"=w681:errorcluster)  [unwired: 8 in, 1 out]
      n220 = for {
        shift-right: [w765] -> w679
        shift-left: string[][] [] ("DCPowerInfoArray") -> [w766]
        tunnel: w669 -> [w781] mode=indexing
        shift-right: [w750] -> w655
        shift-left: w681 -> [w757]
        shift-right: [w758] -> w662
        shift-left: w663 -> [w758]
        shift-right: [w759] -> w664
        shift-left: w665 -> [w759]
        shift-right: [w760] -> w666
        shift-left: w667 -> [w760]
        shift-right: [w761] -> w668
        shift-left: w669 -> [w761]
        shift-right: [w762] -> w654
        shift-left: w670 -> [w762]
        shift-right: [w763] -> w671
        shift-left: w672 -> [w763]
        shift-right: [w764] -> w673
        shift-left: w674 -> [w764]
        n221 = Unbundle(w781) -> ("VISA resource name"=w780:refnum<visa-resource-name>, "Frequency (GHz) Output"=w774:dbl, "Power (dBm) Output"=w771:dbl)  [unwired: 2 out]
        n222 = Decimal String To Number(string="8") -> (number=w769:i32)  [unwired: 2 in, 1 out]
        n223 = VISA Write(VISA resource name=w780, write buffer="*IDN?", error in (no error)=w757) -> (VISA resource name out=w776:refnum<visa-resource-name>, return count=w778:u32, error out=w782:errorcluster)
        n224 = Number To Fractional String(number=w771, precision (6)=w769) -> (F-format string=w772:string)  [unwired: 2 in]
        n225 = Add(x=w778, y=u32 10) -> (x+y=w775:u32)
        n226 = Number To Fractional String(number=w774, precision (6)=w769) -> (F-format string=w773:string)  [unwired: 2 in]
        n227 = VISA Read(VISA resource name=w776, byte count=w775, error in (no error)=w782) -> (read buffer=w756:string, error out=w751:errorcluster)  [unwired: 2 out]
        n228 = Search and Replace String(replace all?=TRUE ("replace all? (F)"), input string=w756, search string=",", replace string="_" ("replace string (\"\")"), error in=w751) -> (result string=w753:string, error out=w750:errorcluster)  [unwired: 3 in, 2 out]
        n229 = Build Array(w753, w773, w772) -> (w768:string[])
        n230 = Insert Into Array(array=w766, index (col)=0 ("index (row)"), new element=w768) -> (w765:string[][])  [unwired: 1 in]
      }
      n231 = Build Array("Instrument Name", "Frequency (GHz)" ("element"), "Power (dBm)" ("element")) -> (w675:string[])
      n232 = Build Path(base path=w599, name or relative path="RFSource_Params.csv") -> (appended path=w660:path)
      n233 = Insert Into Array(array=w679, index (col)=0 ("disabled index (col)"), new element=w675) -> (w656:string[][])  [unwired: 1 in]
      n234 = call-poly <vilib>:"Write Delimited Spreadsheet.vi"("file path (dialog if empty)"=w660, "format (%s)"="%s" ("format (%.3f)"), "2D data"=w656, "error in (no error)"=w655, "transpose? (no:F)"=TRUE, "delimiter (\\t)"="," ("delimiter (\\t)")) -> ("error out"=w635:errorcluster)  [unwired: 8 in, 1 out]
      n235 = Strip Path(path=w599) -> (name=w653:string)  [unwired: 1 out]
      n236 = Unbundle(w654) -> ("DUT"=w652:string, "Ion (ex Kr)"=w651:string, "Board Number"=w650:string, "Effective LET"=w649:string, "Test Type"=w648:T16)  [unwired: 1 out]
      n237 = case shown="\"Single Event Latchup\", Default" w648 {
        tunnel: ["Single Event Latchup (SEL)" "Single Event Transient (SET)"] -> w647
        frame "Single Event Latchup", Default {
        }
        frame "Single Event Transient" {
        }
      }
      n238 = Build Array("Run Number" ("name"), "DUT" ("element"), "Ion" ("element"), "Board Number" ("element"), "Effective LET" ("element"), "Test Type" ("element")) -> (w646:string[])
      n239 = Build Array(w653, w652, w651, w650, w649, w647) -> (w645:string[])
      n240 = Build Array(w646, w645) -> (w634:string[][])
      n241 = Build Path(base path=w599, name or relative path="RunData_Params.csv") -> (appended path=w640:path)
      n242 = call-poly <vilib>:"Write Delimited Spreadsheet.vi"("file path (dialog if empty)"=w640, "format (%s)"="%s" ("format (%.3f)"), "2D data"=w634, "error in (no error)"=w635, "transpose? (no:F)"=TRUE, "delimiter (\\t)"="," ("delimiter (\\t)")) -> ()  [unwired: 8 in, 2 out]
      n243 = List Folder(path=w599, pattern="*NULL.txt") -> (path out=w618:path, filenames=w619:string[], error out=w620:errorcluster)  [unwired: 2 in, 1 out]
      n244 = for {
        tunnel: [w735] -> w630
        tunnel: w618 -> [w735]
        tunnel: w619 -> [w737] mode=indexing
        shift-right: [w738] -> w621
        shift-left: w620 -> [w739]
        n245 = Build Path(base path=w735, name or relative path=w737) -> (appended path=w736:path)
        n246 = Delete(path (use dialog)=w736, error in=w739) -> (error out=w738:errorcluster)  [unwired: 3 in, 2 out]
      }
      n247 = Get Date/Time String(date format (0)=enum16{"short", "long", "abbreviated"}."short", seconds (now)=w600, want seconds? (F)=TRUE) -> (date string=w624:string, time string=w623:string)
      n248 = Concatenate Strings(w624, "_" ("string"), w623) -> (w625:string)
      n249 = Strip Path(path=w630) -> (name=w616:string)  [unwired: 1 out]
      n250 = Build Path(base path=w630, name or relative path="BeginRecordTimeStamp.txt") -> (appended path=w631:path)
      n251 = Concatenate Strings(w616, "_DCPOWER_COPYFOLDER" ("name or relative path")) -> (w617:string)
      n252 = Open/Create/Replace File(file path (use dialog)=w631, error in=w621, operation (0:open)=T15."open or create", access (0:read/write)=enum16{"read/write", "read-only", "write-only"}."read/write") -> (refnum out=w626:refnum<file>, error out=w622:errorcluster)  [unwired: 2 in, 1 out]
      n253 = Build Path(base path=w630, name or relative path=w617) -> (appended path=w610:path)
      n254 = Write to Text File(file (use dialog)=w626, text=w625, error in=w622) -> (refnum out=w628:refnum<file>, error out=w627:errorcluster)  [unwired: 1 in, 1 out]
      n255 = Close File(refnum=w628, error in=w627) -> (error out=w629:errorcluster)  [unwired: 1 out]
      n256 = Create Folder(path (use dialog)=w610, error in=w629) -> (created path=w614:path, error out=w611:errorcluster)  [unwired: 1 in, 1 out]
      n257 = List Folder(path=w630, error in=w611) -> (path out=w612:path, filenames=w613:string[], error out=w615:errorcluster)  [unwired: 2 in, 1 out]
      n258 = for {
        tunnel: w612 -> [w745]
        tunnel: w613 -> [w744] mode=indexing
        tunnel: w614 -> [w740]
        shift-right: [w747] -> w601
        shift-left: w615 -> [w741]
        tunnel: [w740] -> _
        n259 = Build Path(base path=w745, name or relative path=w744) -> (appended path=w742:path)
        n260 = Build Path(base path=w740, name or relative path=w744) -> (appended path=w743:path)
        n261 = Copy(8:w741, 9:TRUE ("overwrite (F)"), 10:w743, 11:w742) -> (0:w747:errorcluster)  [unwired: 1 in, 2 out]
      }
    }
  }
  "VISAPowerInfoInputOutput" <- w42
  "Run Data SubPanel Output" <- w44
  "Data Was Collected?" <- w38
  "DCPowerInfoArray" <- w37
  "OscilloscopeInfoArray" <- w12
  "RFSourceInfoArray" <- w27
  "RF Subpanel Output" <- w46
  "error out" <- w15
  "Oscilloscope Info Array" <- w11
  "DCPowerInformationClusterArray_Output" <- w5
